vi "gas sensor with thinkspeak.vi"() -> ()   [LabVIEW 2017]
uses:
  <vilib>/httpClient/LabVIEWHTTPClient.lvlib
panel:
  in  "error in (no error)":errorcluster
  in  "initial string":string
  out "body":string
  out "headers":string
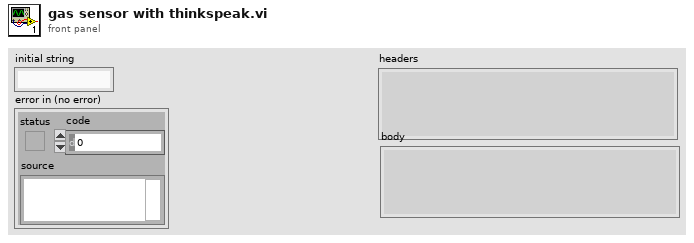
[diagram p1: front panel]
types:
  T1 = typedef "LabVIEWHTTPClient.lvlib/ClientHandle.ctl" = refnum<k1>
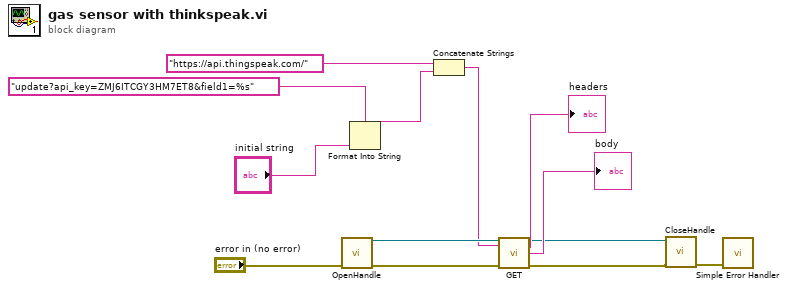
[diagram p0: block diagram]
diagram:
  n1 = call <vilib>:"OpenHandle.vi"("error in (no error)"="error in (no error)") -> ("client handle out"=w8:T1, "error out"=w9:errorcluster)  [unwired: 13 in]
  n2 = Format Into String(format string="update?api_key=ZMJ6ITCGY3HM7ET8&field1=%s", "initial string") -> (resulting string=w4:string)  [unwired: 2 in, 1 out]
  n3 = Concatenate Strings("https://api.thingspeak.com/" ("string"), w4) -> (w3:string)
  n4 = call <vilib>:"GET.vi"("client handle"=w8, "url"=w3, "error in (no error)"=w9) -> ("client handle out"=w11:T1, "headers"=→"headers":string, "body"=→"body":string, "error out"=w10:errorcluster)  [unwired: 9 in]
  n5 = call <vilib>:"CloseHandle.vi"("client handle"=w11, "error in (no error)"=w10) -> ("error out"=w7:errorcluster)  [unwired: 13 in]
  n6 = call <vilib>:"Simple Error Handler.vi"("error in (no error)"=w7) -> ()  [unwired: 4 in, 5 out]
